vi "FTW-Producer-Worker.vi"(1 "Shutdown Notification":refnum<notifier>, 2 "Endpoint Type":refnum<class "FTW-Endpoint.lvclass">, 3 "Address":string, 4 "Pipe":refnum<queue>) -> ()   [LabVIEW 2013, in "FTW-Producer.lvclass"]
uses:
  FTW-Producer.lvclass
  Endpoint/FTW-Endpoint.lvclass
panel:
  out "connected":bool
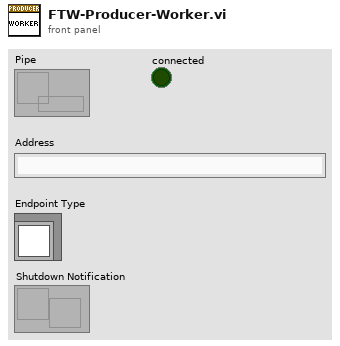
[diagram p1: front panel]
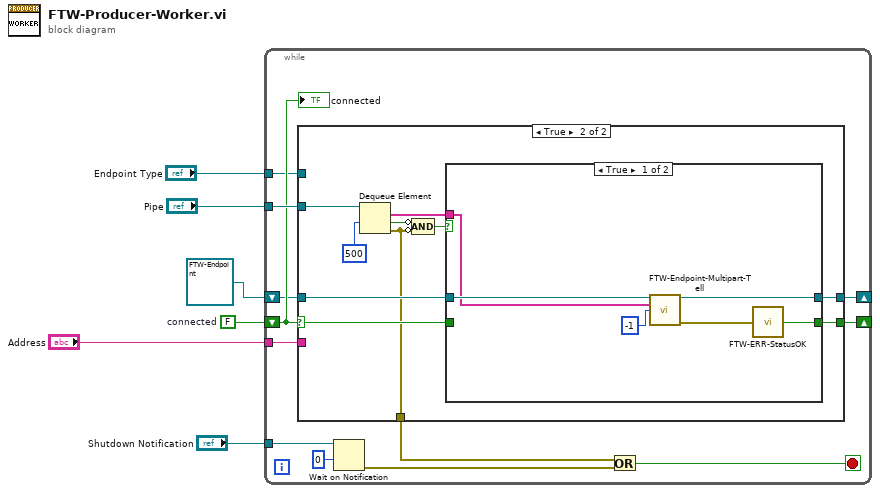
[diagram p0: block diagram]
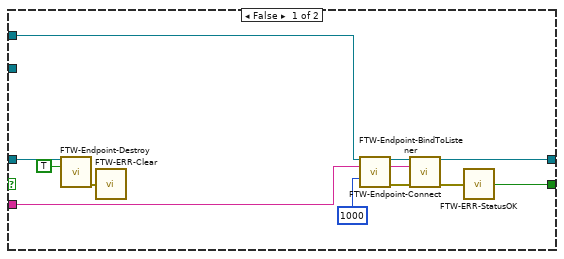
[diagram p2: hidden frame]
diagram:
  w5 = FALSE  # connected
  n1 = while {
    tunnel: "Pipe" -> [w18]
    shift-right: [w14] -> _
    shift-left: w5 -> [w17]
    shift-right: [w15] -> _
    shift-left: refnum<class "FTW-Endpoint.lvclass"> refnum ("FTW Endpoint") -> [w10]
    tunnel: "Address" -> [w16]
    tunnel: "Shutdown Notification" -> [w12]
    tunnel: "Endpoint Type" -> [w7]
    stop <- w9 stop-if-true
    n2 = case shown="True" w17 {
      selector: w17 -> [_ w33]
      tunnel: w18 -> [_ w40]
      tunnel: w16 -> [w27 _]
      tunnel: [w26 w37] -> w15
      tunnel: [w25 w34] -> w14
      tunnel: w10 -> [w22 w38]
      tunnel: [_ w31] -> w8
      tunnel: w7 -> [w19 _]
      frame False {
        n3 = call-dynamic "FTW-Endpoint-Destroy.vi"("FTW Endpoint"=w22, "Force Destroy"=TRUE) -> ("error out"=w20:errorcluster)  [unwired: 13 in]
        n4 = call "FTW-ERR-Clear.vi"("error to snuff"=w20) -> ()  [unwired: 1 out]
        n5 = call-dynamic "FTW-Endpoint-BindToListener.vi"("FTW-Endpoint In"=w19, "Address"=w27, "Timeout"=1000) -> ("FTW-Endpoint Out"=w30:refnum<class "FTW-Endpoint.lvclass">, "Actual Address"=w28:string, "error out"=w29:errorcluster)  [unwired: 10 in]
        n6 = call-dynamic "FTW-Endpoint-Connect.vi"("FTW Endpoint"=w30, "Endpoint Address"=w28, "error in"=w29) -> ("FTW Endpoint out"=w26:refnum<class "FTW-Endpoint.lvclass">, "error out"=w24:errorcluster)  [unwired: 11 in]
        n7 = call "FTW-ERR-StatusOK.vi"("error to check"=w24) -> ("Status OK?"=w25:bool)
      }
      frame True {
        n8 = Dequeue Element(queue=w40, timeout in ms (-1)=500 ("Timeout")) -> (element=w32:string[], timed out?=w36:bool, error out=w31:errorcluster)  [unwired: 1 in, 1 out]
        n9 = Compound Arithmetic op=AND(invert w36, invert w31) -> (w35:bool)
        n10 = case shown="True" w35 {
          tunnel: w38 -> [w46 w48]
          tunnel: [w45 w48] -> w37
          tunnel: w32 -> [w42 _]
          tunnel: [w43 w47] -> w34
          tunnel: w33 -> [_ w47]
          frame True {
            n11 = call-dynamic "FTW-Endpoint-Multipart-Tell.vi"("FTW Endpoint"=w46, "Multipart Message"=w42, "Timeout"=-1) -> ("FTW Endpoint out"=w45:refnum<class "FTW-Endpoint.lvclass">, "error out"=w44:errorcluster)  [unwired: 10 in, 1 out]
            n12 = call "FTW-ERR-StatusOK.vi"("error to check"=w44) -> ("Status OK?"=w43:bool)
          }
          frame False {
          }
        }
      }
    }
    n13 = Wait on Notification(notifier=w12, timeout in ms (-1)=0) -> (error out=w11:errorcluster)  [unwired: 2 in, 3 out]
    n14 = Or(x=w8, y=w11) -> (x .or. y?=w9:bool)
    "connected" <- w17
  }
